vi "databaseTesting with Saphire DB VI.vi"() -> ()   [LabVIEW 2017]
uses:
  <vilib>/SAPHIR/GDataBase for MySQL(tm)/MySQL/public/controls/ClientAuthentication.ctl
  <vilib>/SAPHIR/GDataBase for MySQL(tm)/MySQL/MySQLConnector.lvclass
panel:
  out "Image":T1(plugin-control)
  in  "File Path":path=path "C:/Users/OmerLab/Documents/GitHub/RamanSpecUsingStageXY/imagesForTesting/Snap-15.jpg"
  out "Core Pressure":dbl[](graph)
  out "Core Temperature":dbl[](graph)
  out "max pressure value":dbl format="%#.6g"
  out "min pressure value":dbl format="%#.6g"
  out "max temperature value":dbl format="%#.6g"
  out "min temperature value":dbl format="%#.6g"
  in  "Stop":bool
  out "Number of Records":i32
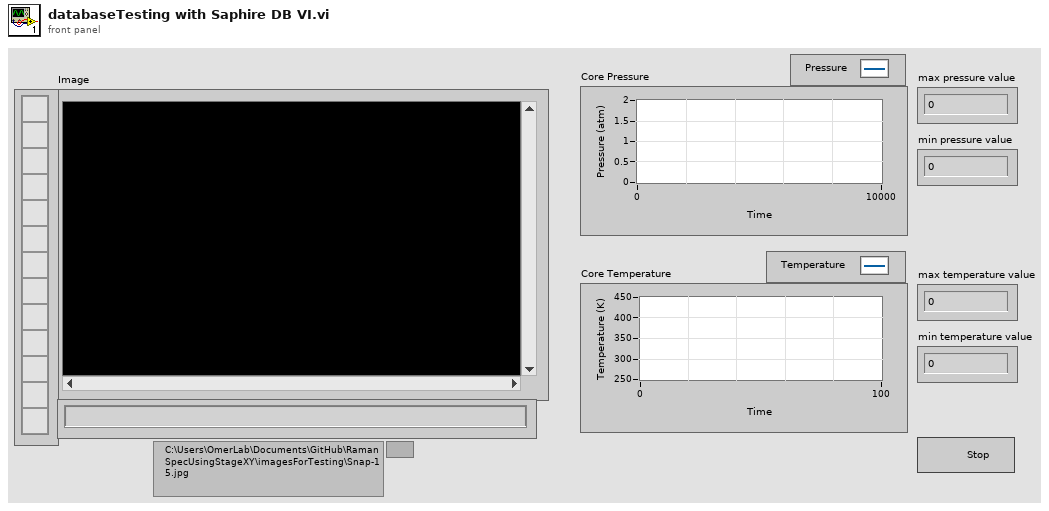
[diagram p1: front panel]
types:
  T1 = typedef "IMAQ Image.ctl" = refnum<image>
  T2 = cluster{"RunNumber":i32, "CorePressure":dbl[], "MaxPressureValue":dbl, "MinPressureValue":dbl, "CoreTemperature":dbl[], "MaxTemperatureValue":dbl, "MinTemperatureValue":dbl}
  T3 = typedef "MySQLVIEW.lvlib/MySQLConnector.lvclass/ClientAuthentication.ctl" = cluster{"username":string, "password":string, "database":string}
  T4 = typedef "Image Type" = u32
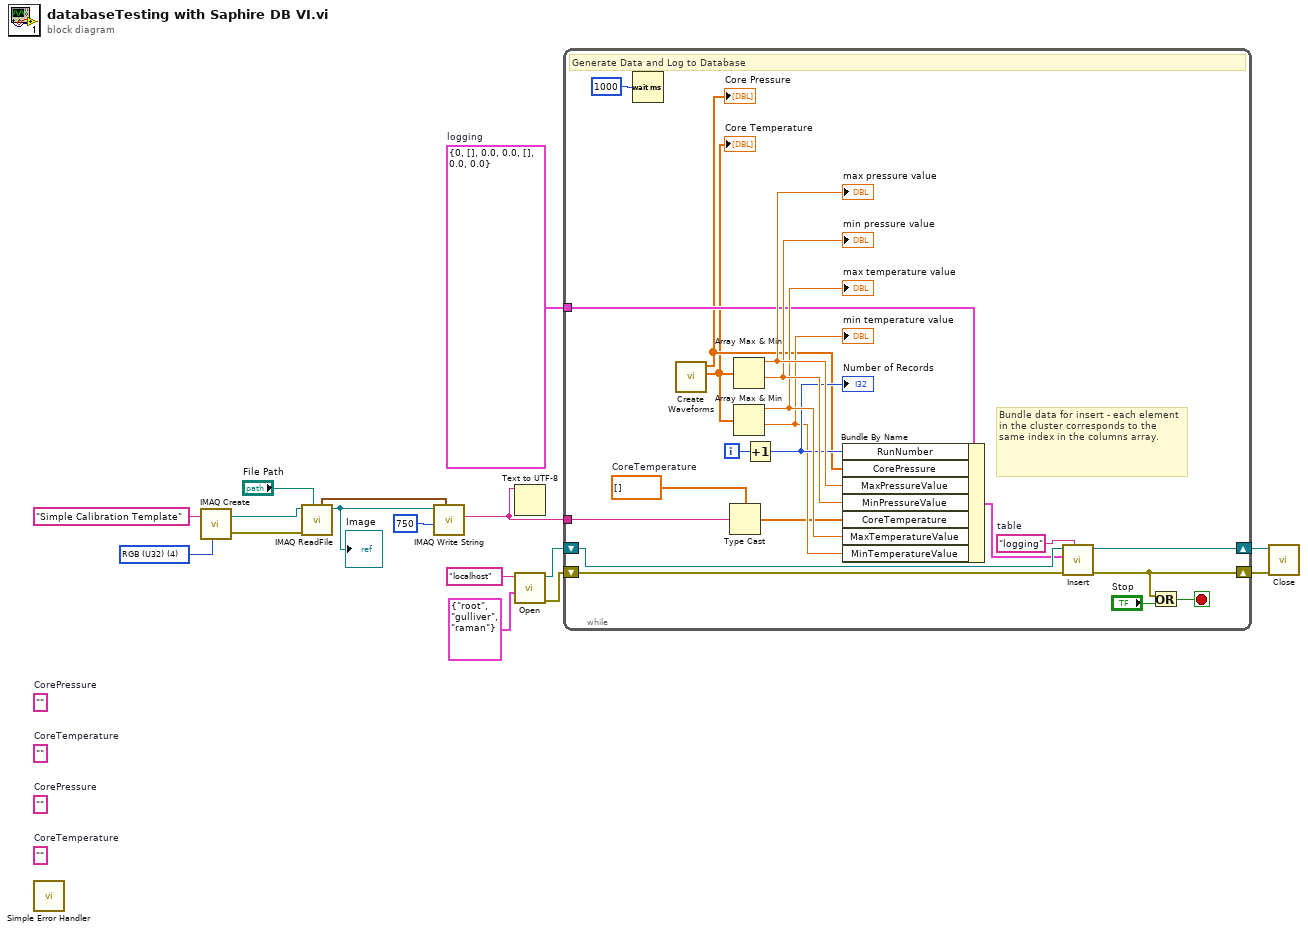
[diagram p0: block diagram]
diagram:
  (unwired) ""  # CoreTemperature
  (unwired) ""  # CorePressure
  (unwired) ""  # CoreTemperature
  (unwired) ""  # CorePressure
  w2 = T2 {"RunNumber"=0, "CorePressure"=[], "MaxPressureValue"=0.0, "MinPressureValue"=0.0, "CoreTemperature"=[], "MaxTemperatureValue"=0.0, "MinTemperatureValue"=0.0}  # logging
  w12 = T4 4 items=["Grayscale (U8)", "Grayscale (I16)", "Grayscale (SGL)", "Complex (CSG)", "RGB (U32)", "HSL (U32)", "RGB (U64)", "Grayscale (U16)"] ("Image Type")
  n1 = call <vilib>:"Simple Error Handler.vi"() -> ()  [unwired: 5 in, 5 out]
  n2 = call "IMAQ Create"("Image Name"="Simple Calibration Template", "Image Type"=w12) -> ("New Image"=w14:T1, "error out"=w16:errorcluster)  [unwired: 2 in, 1 out]
  n3 = call "IMAQ ReadFile"("File Path"="File Path", "error in (no error)"=w16, "Image"=w14) -> ("Image Out"=w11:T1, "Color Palette out"=w10:cluster{"Red":u8, "Green":u8, "Blue":u8}[])  [unwired: 4 in, 3 out]
  "Image" <- w11
  n4 = call-poly "IMAQ Write String"("Color Palette"=w10, "Image Quality"=u32 750, "Image"=w11) -> ("FileString"=w1:string)  [unwired: 6 in, 2 out]
  n5 = Text to UTF-8(11:w1) -> ()  [unwired: 2 in, 2 out]
  n6 = call <vilib>:"Open.vi"("clientAuthentication"=T3 {"username"="root", "password"="gulliver", "database"="raman"}, "host"="localhost") -> ("error out"=w5:errorcluster, "MySQL out"=w6:refnum<class "MySQLConnector.lvclass">)  [unwired: 8 in]
  n7 = while {
    shift-right: [w27] -> w3
    shift-left: w5 -> [w26]
    shift-right: [w28] -> w4
    shift-left: w6 -> [w29]
    tunnel: w2 -> [w25]
    tunnel: w1 -> [w20]
    i -> [w34]
    stop <- w32 stop-if-true
    w21 = dbl[] []  # CoreTemperature
    w24 = "logging"  # table
    # "Bundle data for insert - each element in the cluster corresponds to the same index in the columns array."
    # "Generate Data and Log to Database"
    n8 = Wait (ms)(milliseconds to wait=u32 1000) -> ()  [unwired: 1 out]
    n9 = call "Create Waveforms.vi"() -> ("core temperature"=w17:dbl[], "core pressure"=w18:dbl[])  [unwired: 10 in]
    "Core Pressure" <- w18
    "Core Temperature" <- w17
    n10 = Type Cast(type=w21, x=w20) -> (*(type *) &x=w19:dbl[])
    n11 = Array Max & Min(array=w17) -> (max value=w37:dbl, min value=w36:dbl)  [unwired: 2 out]
    "max pressure value" <- w37
    "min pressure value" <- w36
    n12 = Array Max & Min(array=w17) -> (max value=w35:dbl, min value=w23:dbl)  [unwired: 2 out]
    "max temperature value" <- w35
    "min temperature value" <- w23
    n13 = Increment(x=w34) -> (x+1=w31:i32)
    "Number of Records" <- w31
    n14 = Bundle By Name(cluster=w25, "RunNumber"=w31, "CorePressure"=w18, "MaxPressureValue"=w37, "MinPressureValue"=w36, "CoreTemperature"=w19, "MaxTemperatureValue"=w35, "MinTemperatureValue"=w23) -> (w22:T2)
    n15 = call <vilib>:"Insert.vi"("tableName (\"\" : clusterData label)"=w24, "error in (no error)"=w26, "clusterData"=w22, "MySQL in"=w29) -> ("error out"=w27:errorcluster, "MySQL out"=w28:refnum<class "MySQLConnector.lvclass">)  [unwired: 5 in, 1 out]
    n16 = Or(x=w27, y="Stop") -> (x .or. y?=w32:bool)
  }
  n17 = call <vilib>:"Close.vi"("error in (no error)"=w3, "MySQL in"=w4) -> ()  [unwired: 9 in, 1 out]
